vi "Write U32.vi"(7 "key":string, 8 "error in (no error)":errorcluster, 9 "Value":u32, 11 "Configuration File In":refnum<class "Configuration File.lvclass">) -> (0 "error out":errorcluster, 3 "Configuration File Out":refnum<class "Configuration File.lvclass">)   [LabVIEW 2020, in "Configuration File.lvclass"]
doc: "High-level function for reading configuration file data from process class."
uses:
  Configuration File.lvclass
  <vilib>/Utility/config.llb/Write Key (U32).vi
  <vilib>/Utility/config.llb/NI_LVConfig.lvlib
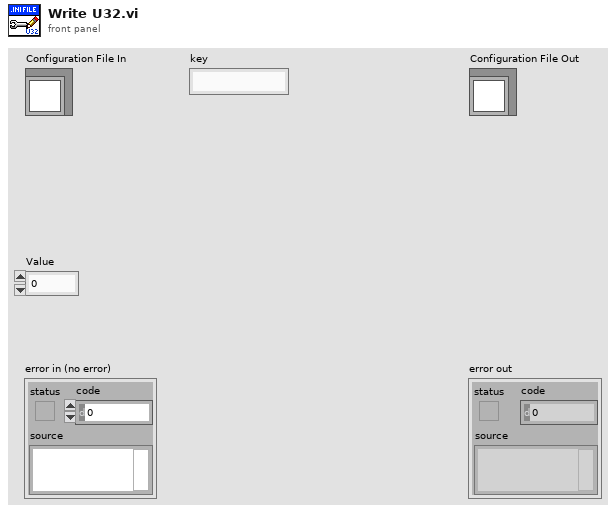
[diagram p1: front panel]
types:
  T1 = typedef "NI_LVConfig.lvlib/Config Data RefNum.ctl" = refnum<k1>
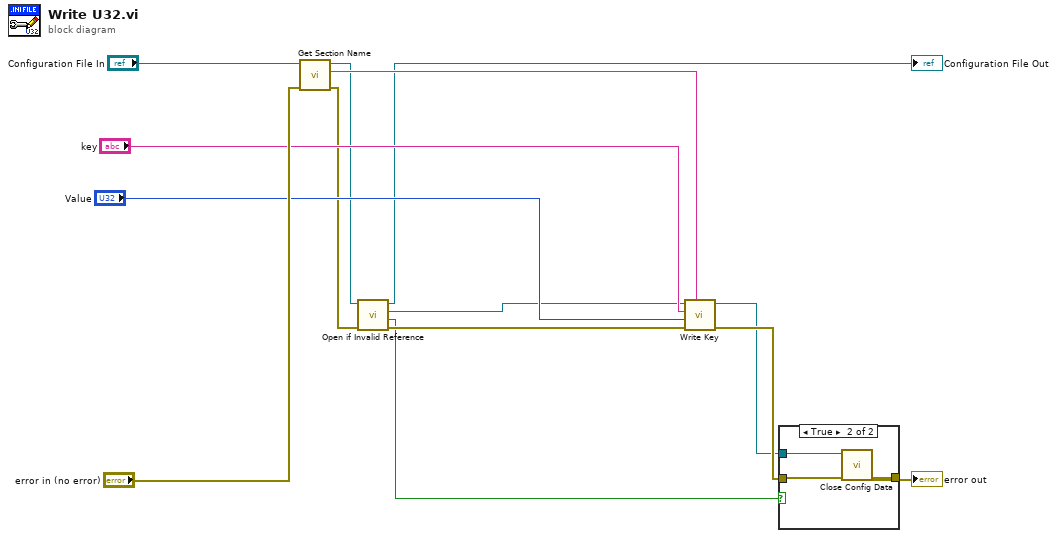
[diagram p0: block diagram]
diagram:
  n1 = call "Get Section Name.vi"("error in (no error)"="error in (no error)", "Configuration File In"="Configuration File In") -> ("error out"=w7:errorcluster, "Section Name"=w10:string, "Configuration File Out"=w9:refnum<class "Configuration File.lvclass">)  [unwired: 7 in]
  n2 = call "Open if Invalid Reference.vi"("error in (no error)"=w7, "Configuration File In"=w9) -> ("error out"=w6:errorcluster, "File opened?"=w1:bool, "refnum out"=w5:T1, "Configuration File Out"=→"Configuration File Out":refnum<class "Configuration File.lvclass">)  [unwired: 6 in]
  n3 = call-poly <vilib>:"Write Key.vi"("section"=w10, "error in (no error)"=w6, "value"="Value", "key"="key", "refnum"=w5) -> ("error out"=w3:errorcluster, "refnum out"=w2:T1)  [unwired: 4 in, 1 out]
  n4 = case shown="True" w1 {
    tunnel: w2 -> [_ w18]
    tunnel: w3 -> [w15 w17]
    tunnel: [w15 w16] -> w4
    frame False {
    }
    frame True {
      n5 = call <vilib>:"Close Config Data.vi"("error in (no error)"=w17, "refnum"=w18) -> ("error out"=w16:errorcluster)  [unwired: 8 in, 1 out]
    }
  }
  "error out" <- w4
